vi "Configure Mask Test (Measurement).vi"(0 "VISA resource name":refnum<visa-resource-name>, 1 "Units (1: Division)":i32(ring)=1 items=["Current", "Division"], 5 "Mask Source (0: Channel 1)":i32(ring) items=["Channel 1", "Channel 2", "Channel 3", "Channel 4"], 7 "Y Delta (0.25 V)":dbl=0.25, 9 "X Delta (0.25 S)":dbl=0.25, 11 "error in (no error)":errorcluster) -> (4 "VISA resource name out":refnum<visa-resource-name>, 15 "error out":errorcluster)   [LabVIEW 2015, in "Agilent 2000 3000 X-Series.lvlib"]
doc: "Configure the measurement settings of mask test."
uses:
  Agilent 2000 3000 X-Series.lvlib
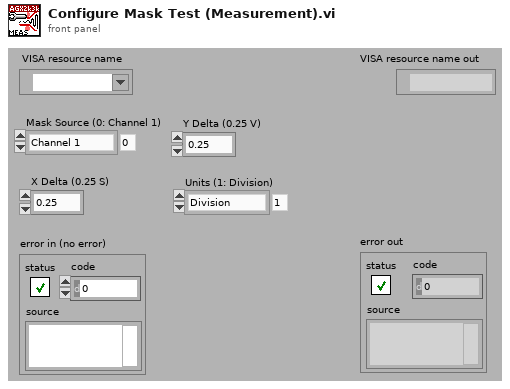
[diagram p1: front panel]
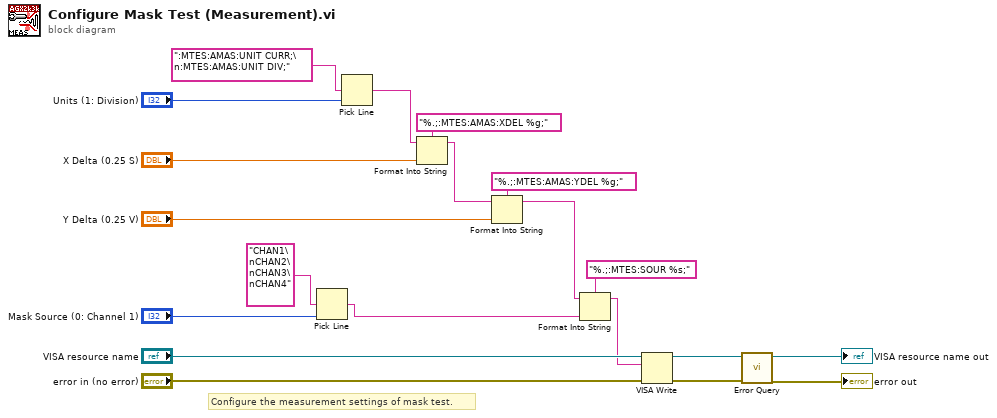
[diagram p0: block diagram]
diagram:
  # "Configure the measurement settings of mask test."
  n1 = Pick Line(multi-line string="CHAN1\nCHAN2\nCHAN3\nCHAN4", line index="Mask Source (0: Channel 1)") -> (output string=w1:string)  [unwired: 1 out]
  n2 = Pick Line(multi-line string=":MTES:AMAS:UNIT CURR;\n:MTES:AMAS:UNIT DIV;", line index="Units (1: Division)") -> (output string=w18:string)  [unwired: 1 out]
  n3 = Format Into String(format string="%.;:MTES:AMAS:XDEL %g;", initial string=w18, "X Delta (0.25 S)") -> (resulting string=w15:string)  [unwired: 1 in, 1 out]
  n4 = Format Into String(format string="%.;:MTES:AMAS:YDEL %g;", initial string=w15, "Y Delta (0.25 V)") -> (resulting string=w5:string)  [unwired: 1 in, 1 out]
  n5 = Format Into String(format string="%.;:MTES:SOUR %s;", initial string=w5, w1) -> (resulting string=w4:string)  [unwired: 1 in, 1 out]
  n6 = VISA Write(VISA resource name="VISA resource name", write buffer=w4, error in (no error)="error in (no error)") -> (VISA resource name out=w10:refnum<visa-resource-name>, error out=w9:errorcluster)  [unwired: 1 out]
  n7 = call "Error Query.vi"("error in (no error)"=w9, "VISA resource name"=w10) -> ("error out"=→"error out":errorcluster, "VISA resource name out"=→"VISA resource name out":refnum<visa-resource-name>)  [unwired: 8 out]
